vi "Tree Menu to String.vi"(11 "Control in":refnum<vi>) -> (3 "delimited string":string)   [LabVIEW 2013, in "main.lvlib"]
uses:
  main.lvlib
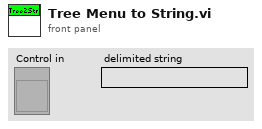
[diagram p1: front panel]
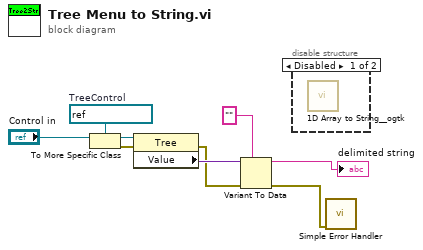
[diagram p0: block diagram]
diagram:
  w7 = refnum<vi> refnum  # TreeControl
  n1 = To More Specific Class(target class=w7, reference="Control in") -> (specific class reference=w8:refnum<vi>, error out=w3:errorcluster)  [unwired: 1 in]
  n2 = property class="Tree"(reference=w8, error in=w3) -> (error out=w2:errorcluster, "Value"=w9:variant)  [unwired: 1 out]
  n3 = Variant To Data(error in=w2, type="", Variant=w9) -> (data=→"delimited string":string, error out=w1:errorcluster)
  n4 = disable-structure shown="Disabled" {
    frame Disabled {
      n5 = call <userlib>:"1D Array to String__ogtk.vi"() -> ()  [unwired: 11 in, 1 out]
    }
    frame Enabled {
    }
  }
  n6 = call <vilib>:"Simple Error Handler.vi"("error in (no error)"=w1) -> ()  [unwired: 4 in, 5 out]
